vi "Static VI.vi"(0 "添加的数组":string[][](array[string])=[["输出电压", "*", "0", "*", "OK"], ["输出电流", "*", "0", "*", "OK"], ["输出功率", "*", "0", "*", "OK"]], 2 "Max":string[](array[string]), 3 "Min":string[](array[string]), 4 "板数":i32, 5 "error in (no error)":errorcluster, 6 "INPUTSTRING":string[](array[string]), 7 "是否为字符串对比":bool, 9 "SQ":string) -> (14 "P/F":bool[](array[boolean]), 16 "SQ out":string[](array[string]), 18 "arrauy out":string[][](array[string]), 19 "error out":errorcluster)   [LabVIEW 2018]
panel:
  out "子数组":string[](array[string])
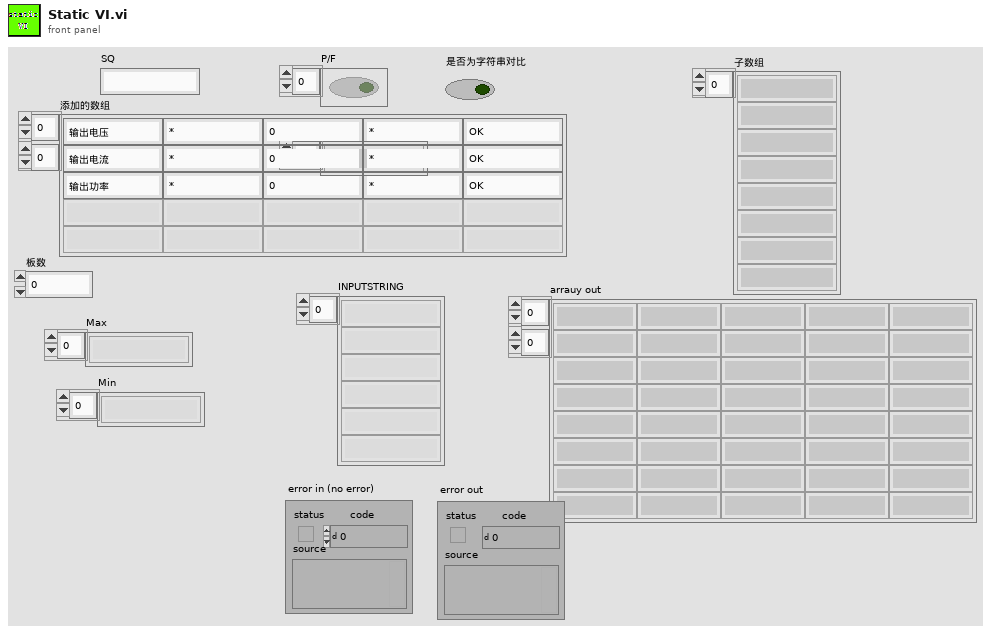
[diagram p1: front panel]
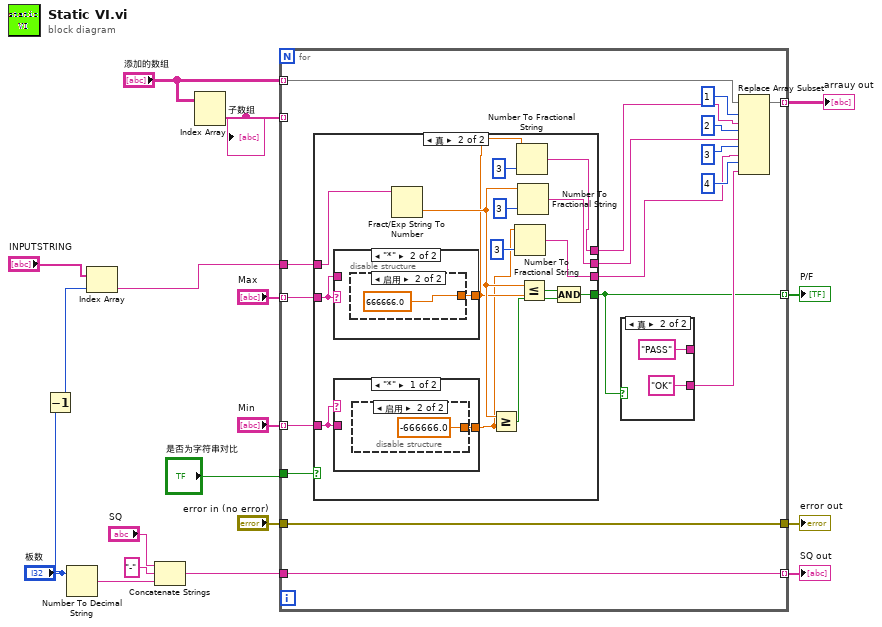
[diagram p0: block diagram]
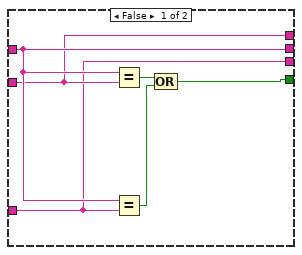
[diagram p2: hidden frame]
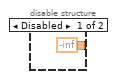
[diagram p3: hidden frame]
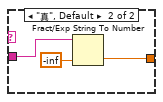
[diagram p4: hidden frame]
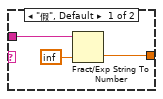
[diagram p5: hidden frame]
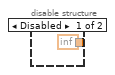
[diagram p6: hidden frame]
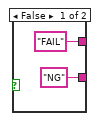
[diagram p7: hidden frame]
diagram:
  n1 = Decrement(x="板数") -> (x-1=w1:i32)
  n2 = Number To Decimal String(number="板数") -> (decimal integer string=w11:string)  [unwired: 1 out]
  n3 = Index Array(array="INPUTSTRING", index=w1) -> (element=w3:string)
  n4 = Concatenate Strings("SQ", "-" ("y"), w11) -> (w10:string)
  n5 = Index Array(array="添加的数组") -> (element=w5:string[])  [unwired: 2 in]
  "子数组" <- w5
  n6 = for {
    tunnel: "添加的数组" -> [w21] mode=indexing
    tunnel: "Max" -> [w24] mode=indexing
    tunnel: "Min" -> [w27] mode=indexing
    tunnel: [w29] -> w17 mode=indexing
    tunnel: [w25] -> w18 mode=indexing
    tunnel: [w28] -> w16 mode=indexing
    tunnel: w10 -> [w28]
    tunnel: "error in (no error)" -> [w26]
    tunnel: [w26] -> w8
    tunnel: "是否为字符串对比" -> [w22]
    tunnel: w3 -> [w23]
    tunnel: w5 -> [_] mode=indexing
    n7 = case shown="真" w22 {
      tunnel: [w38 w56] -> w31
      tunnel: w24 -> [w37 w55]
      tunnel: w27 -> [w36 w54]
      tunnel: [w39 w51] -> w25
      tunnel: w23 -> [w38 w50]
      tunnel: [w37 w43] -> w20
      tunnel: [w36 w42] -> w19
      frame False {
        n8 = Equal?(x=w38, y=w37) -> (x = y?=w41:bool)
        n9 = Equal?(x=w38, y=w36) -> (x = y?=w40:bool)
        n10 = Compound Arithmetic op=OR(w41, w40) -> (w39:bool)
      }
      frame True {
        n11 = case shown="\"*\"" w55 {
          tunnel: w55 -> [w65 _]
          tunnel: [w63 w66] -> w45
          frame "假", Default {
            n12 = Fract/Exp String To Number(string=w65, default (0 dbl)=inf) -> (number=w63:dbl)  [unwired: 3 out]
          }
          frame "*" {
            n13 = disable-structure shown="启用" {
              disable-tunnel: [inf 666666.0] -> w66
              frame Disabled {
              }
              frame Enabled {
              }
            }
          }
        }
        n14 = case shown="\"*\"" w54 {
          tunnel: w54 -> [_ w62]
          tunnel: [w57 w60] -> w44
          frame "*" {
            n15 = disable-structure shown="启用" {
              disable-tunnel: [-inf -666666.0] -> w57
              frame Disabled {
              }
              frame Enabled {
              }
            }
          }
          frame "真", Default {
            n16 = Fract/Exp String To Number(string=w62, default (0 dbl)=-inf) -> (number=w60:dbl)  [unwired: 3 out]
          }
        }
        n17 = Fract/Exp String To Number(string=w50) -> (number=w49:dbl)  [unwired: 1 in, 3 out]
        n18 = Greater Or Equal?(x=w49, y=w44) -> (x >= y?=w52:bool)
        n19 = Number To Fractional String(number=w44, precision (6)=i16 3 ("精度(6)")) -> (F-format string=w42:string)  [unwired: 2 out]
        n20 = Number To Fractional String(number=w45, precision (6)=i16 3 ("精度(6)")) -> (F-format string=w43:string)  [unwired: 2 out]
        n21 = Number To Fractional String(number=w49, precision (6)=i16 3 ("精度(6)")) -> (F-format string=w56:string)  [unwired: 2 out]
        n22 = Less Or Equal?(x=w49, y=w45) -> (x <= y?=w53:bool)
        n23 = Compound Arithmetic op=AND(w53, w52) -> (w51:bool)
      }
    }
    n24 = case shown="真" w25 {
      tunnel: ["NG" "OK"] -> w32
      tunnel: ["FAIL" "PASS"] -> _
      frame False {
      }
      frame True {
      }
    }
    n25 = Replace Array Subset(array=w21, new element #1=w20, index #1=1 ("索引"), new element #2=w31, index #2=2 ("索引"), new element #3=w19, index #3=3 ("索引"), new element #4=w32, index #4=4 ("索引")) -> (w29:string[])
  }
  "P/F" <- w18
  "arrauy out" <- w17
  "SQ out" <- w16
  "error out" <- w8
